vi "Mode Reference.vi"(0 "INL DNL Test in":refnum<class "INL DNL Test.lvclass">, 11 "Error in":errorcluster) -> (4 "INL DNL Test out":refnum<class "INL DNL Test.lvclass">, 6 "VI Refnum":refnum<vi>, 8 "Mode Ref":refnum<vi>, 15 "Error out":errorcluster)   [LabVIEW 2020, in "INL DNL Test.lvclass"]
doc: "Runs the mode page asynchronously."
uses:
  INL DNL Test.lvclass
  Mode Page.vi
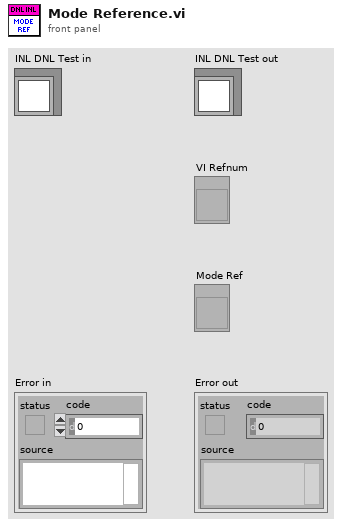
[diagram p1: front panel]
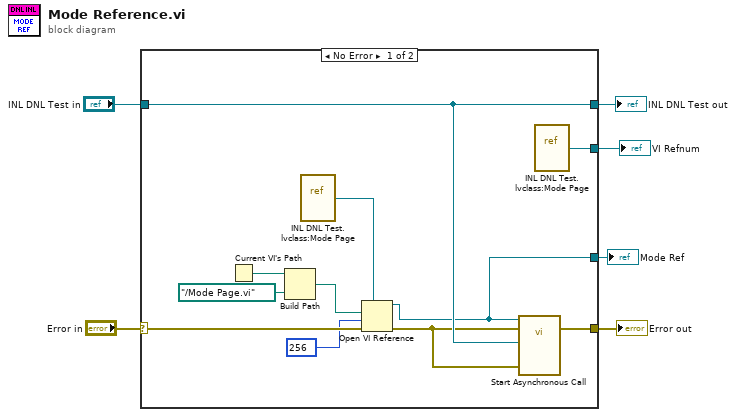
[diagram p0: block diagram]
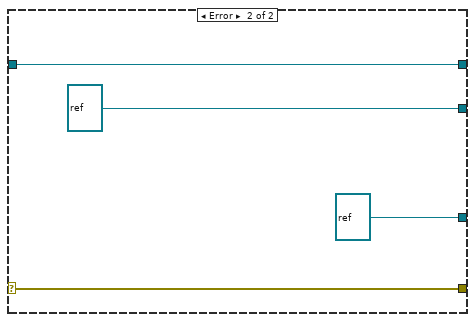
[diagram p2: hidden frame]
diagram:
  n1 = case shown="No Error" "Error in" {
    selector: "Error in" -> [w17 w20]
    tunnel: [w9 w20] -> w5
    tunnel: [w16 refnum<vi> refnum] -> w4
    tunnel: [w10 w21] -> w2
    tunnel: "INL DNL Test in" -> [w10 w21]
    tunnel: [w8 refnum<vi> refnum] -> w1
    frame No Error {
      n2 = Current VI's Path() -> (path=w15:path)
      n3 = Build Path(base path=w15, name or relative path=path "../Mode Page.vi") -> (appended path=w13:path)
      n4 = vi-ref "INL DNL Test.lvclass:Mode Page.vi"() -> (w12:refnum<vi>)
      n5 = Open VI Reference(type specifier VI Refnum (for type only)=w12, vi path=w13, options=256, error in (no error)=w17) -> (vi reference=w8:refnum<vi>, error out=w7:errorcluster)  [unwired: 2 in]
      n6 = call-by-ref "Start Asynchronous Call"(reference=w8, error in=w7, "Error in"=w7, "INL DNL Test in"=w10) -> (error out=w9:errorcluster)  [unwired: 8 in, 3 out]
      n7 = vi-ref "INL DNL Test.lvclass:Mode Page.vi"() -> (w16:refnum<vi>)
    }
    frame Error {
    }
  }
  "Error out" <- w5
  "INL DNL Test out" <- w2
  "VI Refnum" <- w4
  "Mode Ref" <- w1
